vi "Configure 4W Resistance.vi"(0 "VISA resource name":refnum<visa-resource-name>, 1 "Enable Auto Range (T:Enable)":bool=TRUE, 4 "Manual Range (0 Ohm )":dbl format="%.0p", 5 "error in (no error)":errorcluster, 6 "Power Line Cycles (1.00)":dbl=1.0 format="%.2f", 7 "Sampling Interval (0.05)":dbl=0.05 min=0.0002 max=3600.0 step=0.0001 format="%.4f", 12 "Digits (5: 5 1/2)":u16(ring)=5 format="%.0g" items=["3 1/2 Digits"=3, "4 1/2 Digits"=4, "5 1/2 Digits"=5]) -> (14 "VISA resource name out":refnum<visa-resource-name>, 19 "error out":errorcluster)   [LabVIEW 2020, in "ADCMT7451_ADC.lvlib"]
doc: "Configures the measurement type, resolution, and range on the instrument."
uses:
  ADCMT7451_ADC.lvlib
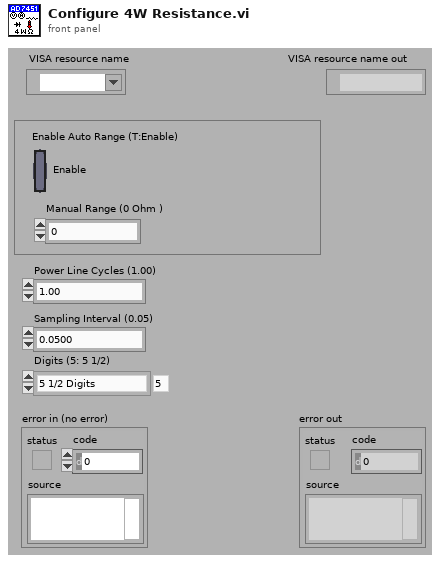
[diagram p1: front panel]
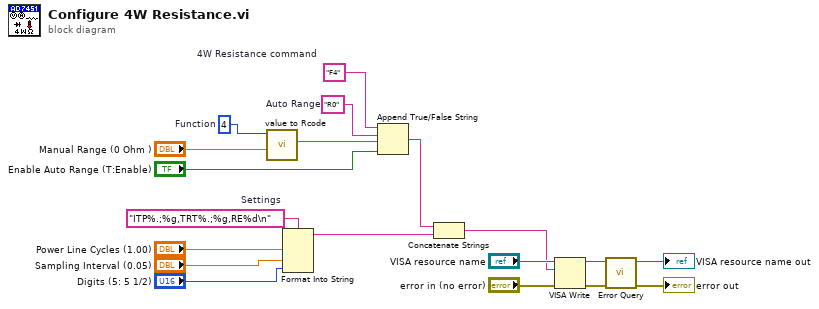
[diagram p0: block diagram]
diagram:
  w3 = "ITP%.;%g,TRT%.;%g,RE%d\n"  # Settings
  w4 = 4  # Function
  w9 = "F4"  # 4W Resistance command
  w12 = "R0"  # Auto Range
  n1 = call "value to Rcode.vi"("Manual Range (0)"="Manual Range (0 Ohm )", "Function (1: DC Volts)"=w4) -> ("Range Set Code"=w6:string)  [unwired: 9 in]
  n2 = Format Into String(format string=w3, "Power Line Cycles (1.00)", "Sampling Interval (0.05)", "Digits (5: 5 1/2)") -> (resulting string=w8:string)  [unwired: 2 in, 1 out]
  n3 = Append True/False String(1:"Enable Auto Range (T:Enable)", 2:w6, 3:w12, 4:w9) -> (0:w11:string)
  n4 = Concatenate Strings(w11, w8) -> (w10:string)
  n5 = VISA Write(VISA resource name="VISA resource name", write buffer=w10, error in (no error)="error in (no error)") -> (VISA resource name out=w15:refnum<visa-resource-name>, error out=w14:errorcluster)  [unwired: 1 out]
  n6 = call "Error Query.vi"("error in (no error)"=w14, "VISA resource name"=w15) -> ("error out"=→"error out":errorcluster, "VISA resource name out"=→"VISA resource name out":refnum<visa-resource-name>)  [unwired: 6 in, 2 out]
